vi "openOptiMOS.vi"(6 "error in (no error)":errorcluster) -> (0 "error out":errorcluster, 2 "cam size":i32[](array[numeric]), 3 "Camera Handle out":u32)   [LabVIEW 2015]
uses:
  LabVIEW/Examples2014_4_3_2_7/Fast Examples/Open-Close Hardware/CamHandle.vi
panel:
  out "Camera open":bool
  # "ExOpenGlobalCam : this subvi opens a camera and stores the handle in a global variable."
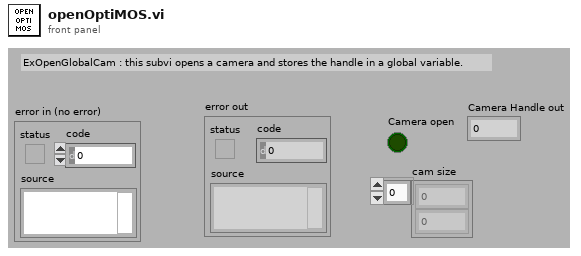
[diagram p1: front panel]
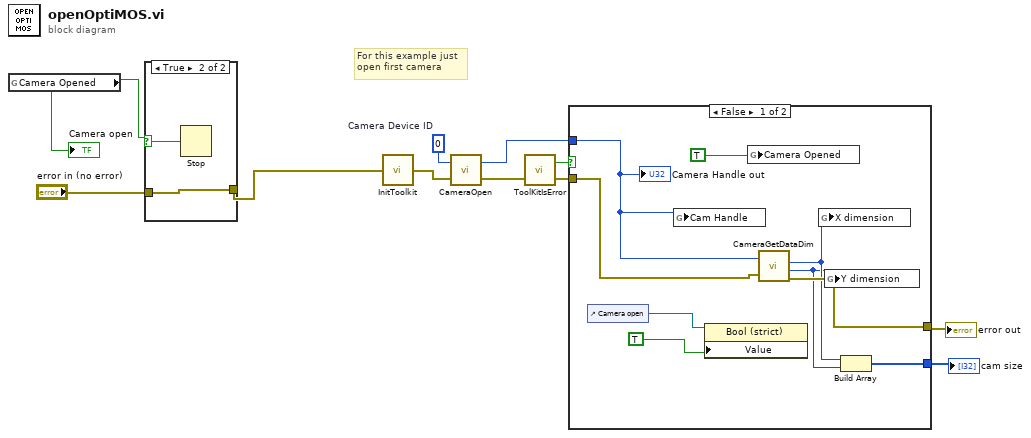
[diagram p0: block diagram]
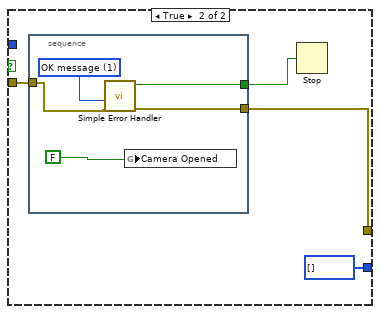
[diagram p3: hidden frame]
diagram:
  w7 = u32 0  # Camera Device ID
  # "For this example just\nopen first camera"
  n1 = global read "CamHandle.vi" "Camera Opened"() -> (w4:bool)
  "Camera open" <- w4
  n2 = case shown="True" w4 {
    selector: w4 -> [_ w13]
    tunnel: [w12 w14] -> w2
    tunnel: "error in (no error)" -> [w12 w14]
    frame False {
    }
    frame True {
      n3 = Stop(stop? (T)=w13) -> ()
    }
  }
  n4 = call <userlib>:"InitToolkit.vi"("error in"=w2) -> ("error out"=w11:errorcluster)
  n5 = call <userlib>:"CameraOpen.vi"("error in"=w11, "Camera Device ID"=w7) -> ("error out"=w10:errorcluster, "Camera Handle"=w6:u32)
  n6 = call <userlib>:"ToolKitIsError.vi"("error in"=w10) -> ("error out"=w8:errorcluster, "Error Flag"=w9:bool)  [unwired: 1 in]
  n7 = case shown="False" w9 {
    tunnel: w8 -> [w22 w27]
    tunnel: [w21 w26] -> w5
    tunnel: w6 -> [w23 _]
    tunnel: [w15 u32[] []] -> w1
    frame False {
      n8 = control-ref of="Camera open"() -> (w18:refnum<vi>)
      n9 = global write "CamHandle.vi" "Cam Handle"(w23) -> ()
      n10 = property class="Bool (strict)"(reference=w18, "Value"=TRUE) -> ()  [unwired: 1 in, 2 out]
      n11 = global write "CamHandle.vi" "Camera Opened"(TRUE) -> ()
      n12 = call <userlib>:"CameraGetDataDim.vi"("Camera Handle"=w23, "error in"=w22) -> ("Xdim"=w17:u32, "Ydim"=w16:u32, "error out"=w21:errorcluster)  [unwired: 1 out]
      n13 = global write "CamHandle.vi" "X dimension"(w17) -> ()
      n14 = global write "CamHandle.vi" "Y dimension"(w16) -> ()
      n15 = Build Array(w17, w16) -> (w15:u32[])
      "Camera Handle out" <- w23
    }
    frame True {
      n16 = stacked-sequence {
        tunnel: w27 -> [w31]
        tunnel: [w30] -> w25
        tunnel: [w29] -> w26
        frame #0 {
          w32 = u16 1 items=["no dialog", "OK message", "continue or stop message"] ("type of dialog (OK msg:1)")
          n17 = call <vilib>:"Simple Error Handler.vi"("type of dialog (OK msg:1)"=w32, "error in (no error)"=w31) -> ("error?"=w30:bool, "error out"=w29:errorcluster)  [unwired: 3 in, 3 out]
          n18 = global write "CamHandle.vi" "Camera Opened"(FALSE) -> ()
        }
      }
      n19 = Stop(stop? (T)=w25) -> ()
    }
  }
  "error out" <- w5
  "cam size" <- w1
